vi "FV-View-R140_txt_multifile.vi"() -> ()   [LabVIEW 2020, in "FV-file_viewer.lvlib"]
uses:
  FV-file_viewer.lvlib
  record_file_handler/VFH-VNA_File_Handler.lvlib
  features/CF-common_features.lvlib
panel:
  out "All Files in Dir":path[](array[path])
  in  "Tab Control":enum32{"Page 1", "Page 3", "Page 2"}(tab)
  in  "Max range":dbl format="%#_6p"
  in  "min range":dbl format="%#_6p"
  out "Ref R":cluster{"Frequency":dbl[], "S21_Imag":dbl[]}[](graph)
  out "Ref I":cluster{"Frequency":dbl[], "S21_Imag":dbl[]}[](graph)
  out "p'":cluster{"Frequency":dbl[], "S21_Imag":dbl[]}[](graph)
  out "p''":cluster{"Frequency":dbl[], "S21_Imag":dbl[]}[](graph)
  in  "Stop":bool
  in  "Max range 2":dbl
  in  "min range 2":dbl
  out "Tan":cluster{"Frequency":dbl[], "S21_Imag":dbl[]}[](graph)
  out "Q [S/m]":cluster{"Frequency":dbl[], "S21_Imag":dbl[]}[](graph)
  in  "Stop 2":bool
  out "appended path":path
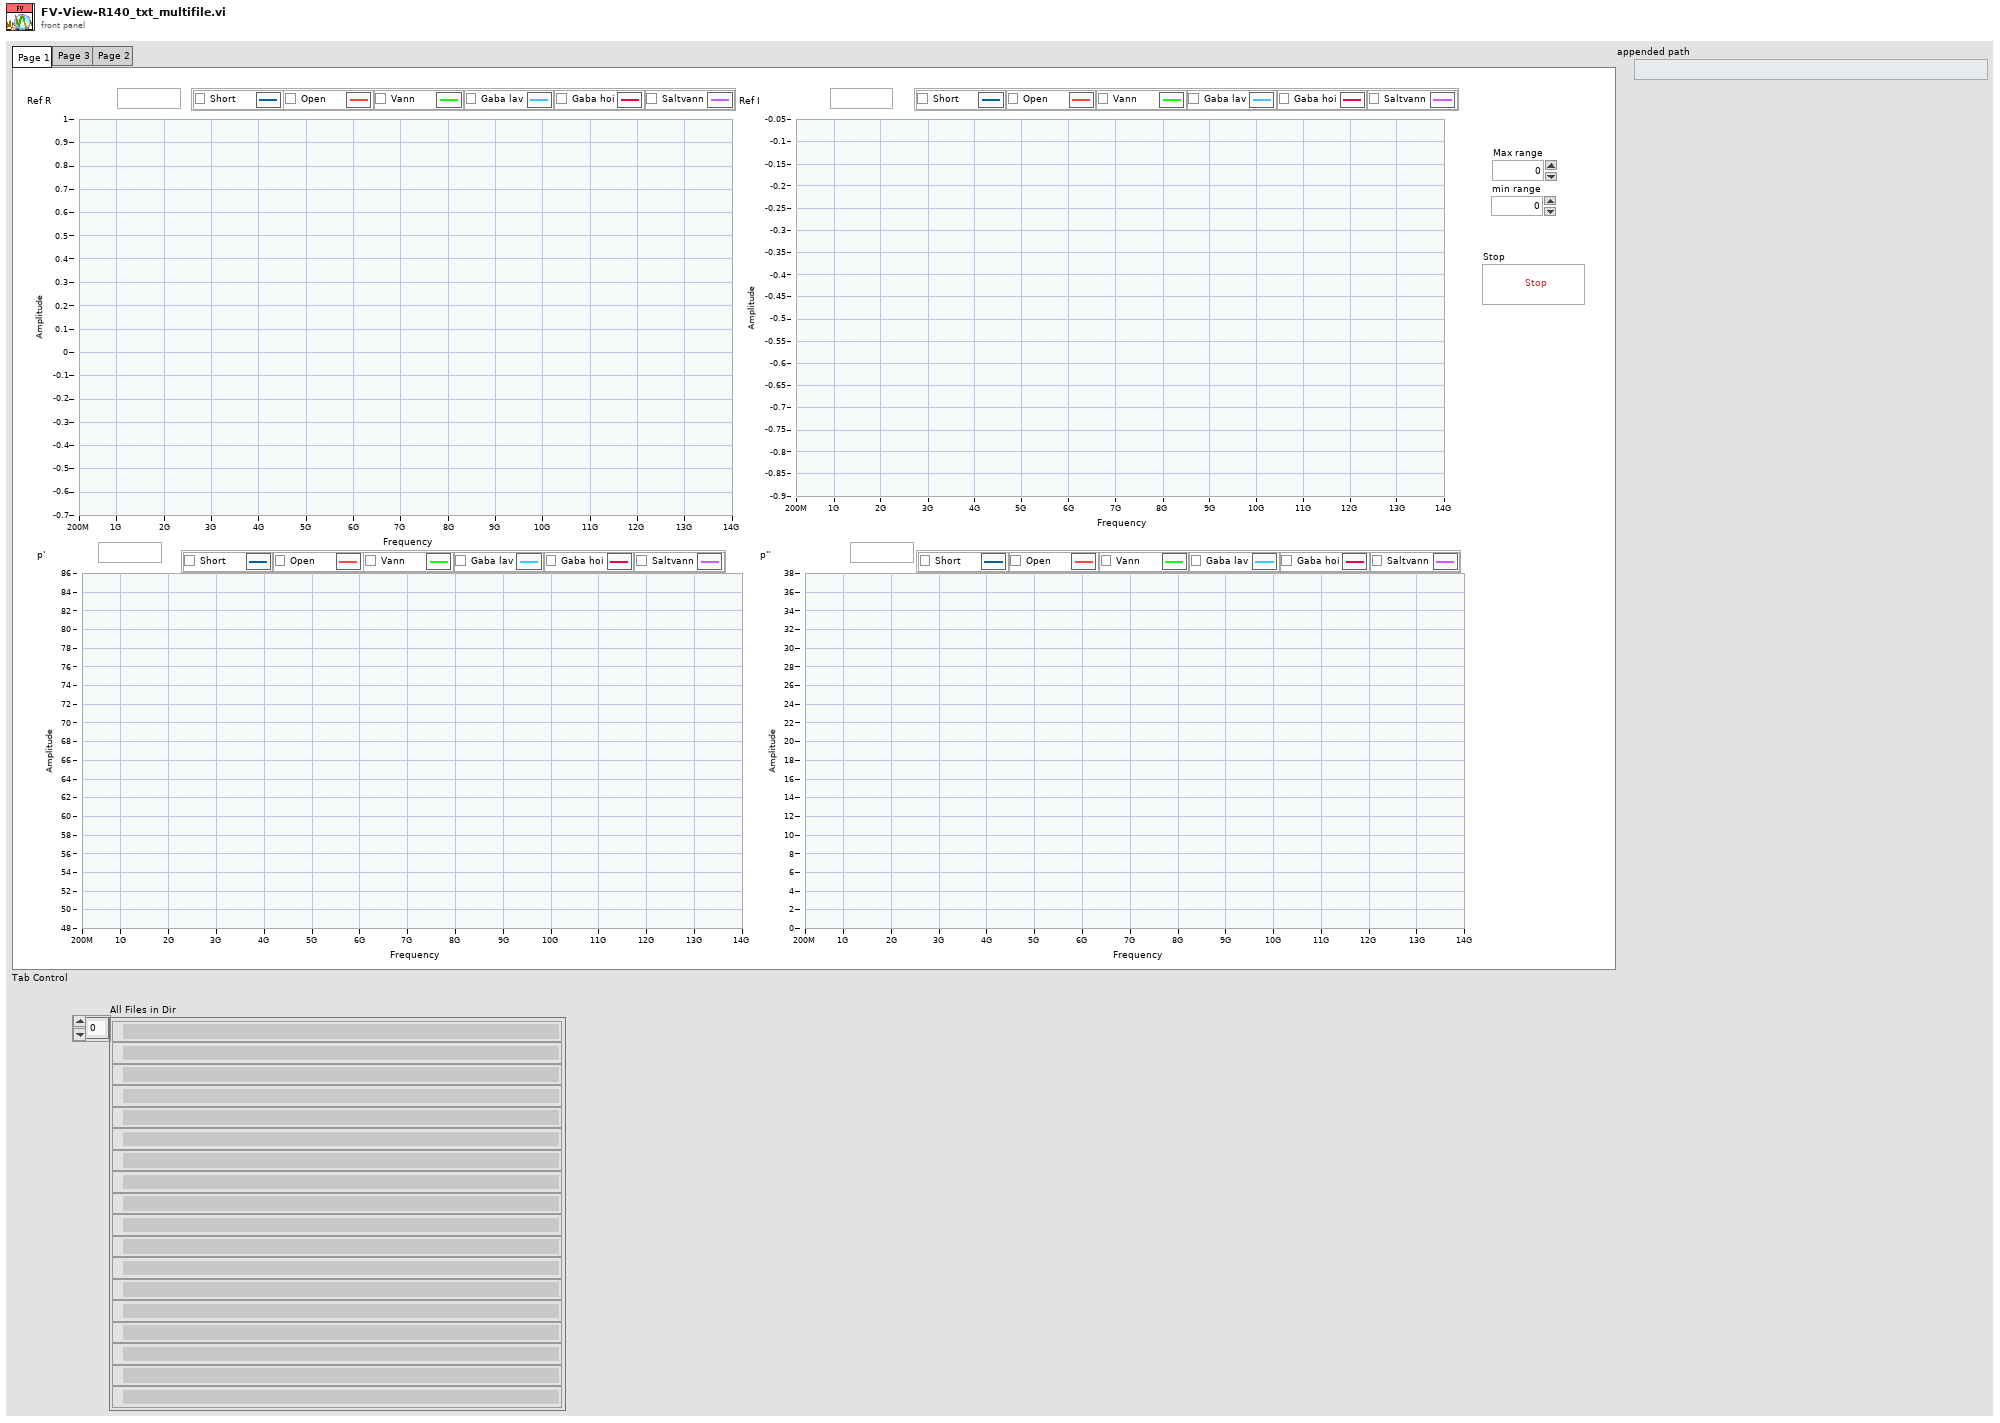
[diagram p1: front panel]
types:
  T1 = typedef "VFH-VNA_File_Handler.lvlib/VFH-file_cluster-LabVIEWVNA.ctl" = cluster{"Frequency":dbl[], "S1_Real":dbl[], "S1_Imag":dbl[], "S11_Real":dbl[], "S11_Imag":dbl[], "S21_Real":dbl[], "S21_Imag":dbl[]}
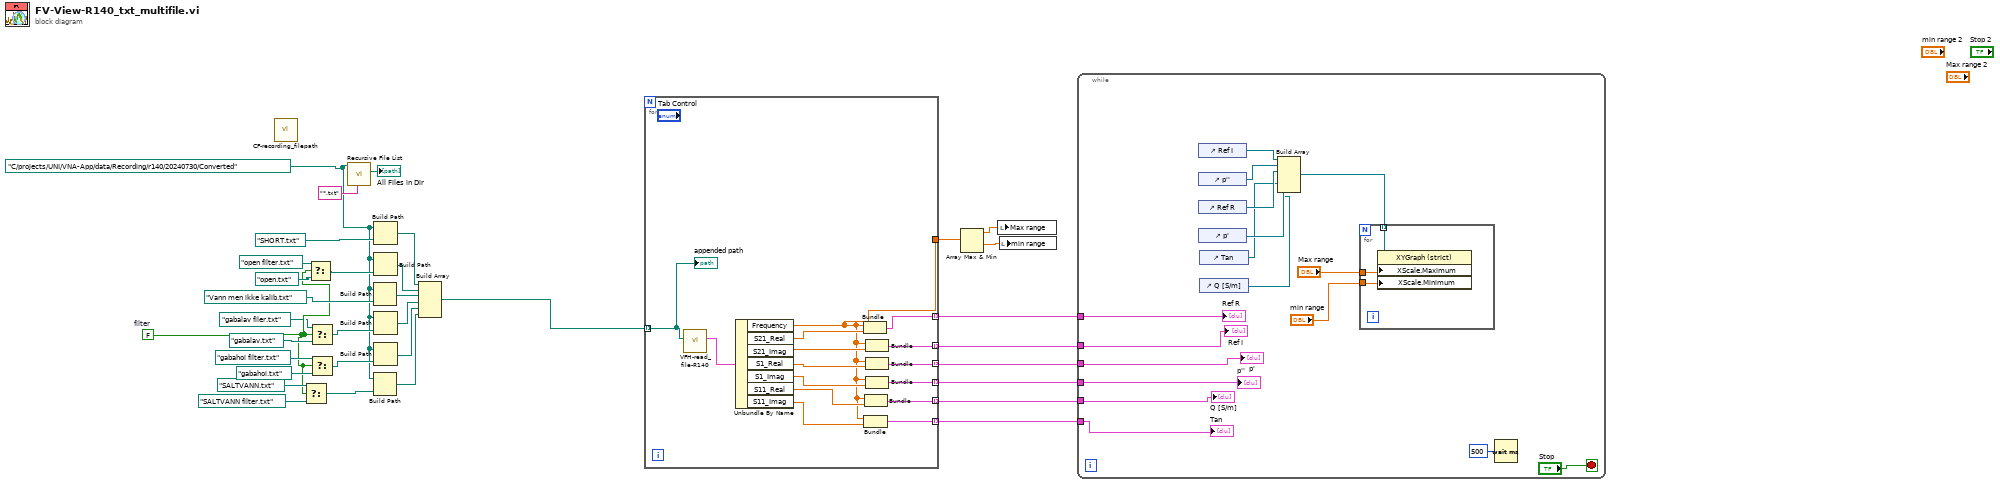
[diagram p0: block diagram]
diagram:
  w6 = FALSE  # filter
  w1 = path "C:/projects/UNI/VNA-App/data/Recording/r140/20240730/Converted" ("Folder Path")
  n1 = call "CF-recording_filepath.vi"() -> ()  [unwired: 10 in, 2 out]
  n2 = Select(t=path "SALTVANN.txt" ("name or relative path"), s=w6, f=path "SALTVANN filter.txt" ("name or relative path")) -> (s? t:f=w10:path)
  n3 = Select(t=path "open filter.txt" ("name or relative path"), s=w6, f=path "open.txt" ("name or relative path")) -> (s? t:f=w8:path)
  n4 = Select(t=path "gabalav filer.txt" ("name or relative path"), s=w6, f=path "gabalav.txt" ("name or relative path")) -> (s? t:f=w5:path)
  n5 = Select(t=path "gabahoi filter.txt" ("name or relative path"), s=w6, f=path "gabahoi.txt" ("name or relative path")) -> (s? t:f=w13:path)
  n6 = call <vilib>:"Recursive File List.vi"("pattern"="*.txt", "Folder Path"=w1) -> ("All Files in Dir"=→"All Files in Dir":path[])  [unwired: 5 in, 4 out]
  n7 = Build Path(base path=w1, name or relative path=path "Vann men ikke kalib.txt") -> (appended path=w23:path)
  n8 = Build Path(base path=w1, name or relative path=w10) -> (appended path=w20:path)
  n9 = Build Path(base path=w1, name or relative path=path "SHORT.txt") -> (appended path=w25:path)
  n10 = Build Path(base path=w1, name or relative path=w8) -> (appended path=w24:path)
  n11 = Build Path(base path=w1, name or relative path=w5) -> (appended path=w22:path)
  n12 = Build Path(base path=w1, name or relative path=w13) -> (appended path=w21:path)
  n13 = Build Array(w25, w24, w23, w22, w21, w20) -> (w18:path[])
  n14 = for {
    tunnel: w18 -> [w36] mode=indexing
    tunnel: [w45] -> w34 mode=indexing
    tunnel: [w44] -> w33 mode=indexing
    tunnel: [w43] -> w32 mode=indexing
    tunnel: [w42] -> w31 mode=indexing
    tunnel: [w39] -> w30
    tunnel: [w38] -> w27 mode=indexing
    tunnel: [w37] -> w26 mode=indexing
    n15 = call "VFH-read_file-R140.vi"("file path (dialog if empty)"=w36) -> ("output cluster"=w35:T1)  [unwired: 9 in, 1 out]
    n16 = Unbundle By Name(w35) -> ("Frequency"=w39:dbl[], "S21_Real"=w49:dbl[], "S21_Imag"=w48:dbl[], "S1_Real"=w47:dbl[], "S1_Imag"=w46:dbl[], "S11_Real"=w40:dbl[], "S11_Imag"=w41:dbl[])
    n17 = Bundle("Frequency"=w39, "S21_Real"=w49) -> (w45:cluster{"Frequency":dbl[], "S21_Real":dbl[]})  [unwired: 1 in]
    n18 = Bundle("Frequency"=w39, "S11_Imag"=w41) -> (w37:cluster{"Frequency":dbl[], "S11_Imag":dbl[]})  [unwired: 1 in]
    n19 = Bundle("Frequency"=w39, "S11_Real"=w40) -> (w38:cluster{"Frequency":dbl[], "S11_Real":dbl[]})  [unwired: 1 in]
    n20 = Bundle("Frequency"=w39, "S21_Imag"=w48) -> (w44:cluster{"Frequency":dbl[], "S21_Imag":dbl[]})  [unwired: 1 in]
    n21 = Bundle("Frequency"=w39, "S1_Real"=w47) -> (w43:cluster{"Frequency":dbl[], "S1_Real":dbl[]})  [unwired: 1 in]
    n22 = Bundle("Frequency"=w39, "S1_Imag"=w46) -> (w42:cluster{"Frequency":dbl[], "S1_Imag":dbl[]})  [unwired: 1 in]
    "appended path" <- w36
  }
  n23 = Array Max & Min(array=w30) -> (max value=w29:dbl, min value=w28:dbl)  [unwired: 2 out]
  n24 = local write "Max range"(w29) -> ()
  n25 = local write "min range"(w28) -> ()
  n26 = while {
    tunnel: w34 -> [w64]
    tunnel: w33 -> [w63]
    tunnel: w32 -> [w62]
    tunnel: w31 -> [w61]
    tunnel: w27 -> [w53]
    tunnel: w26 -> [w52]
    stop <- "Stop" stop-if-true
    n27 = control-ref of="Ref I"() -> (w60:refnum<vi>)
    n28 = control-ref of="p''"() -> (w59:refnum<vi>)
    n29 = control-ref of="Ref R"() -> (w58:refnum<vi>)
    n30 = control-ref of="p'"() -> (w57:refnum<vi>)
    n31 = control-ref of="Tan"() -> (w51:refnum<vi>)
    n32 = control-ref of="Q [S/m]"() -> (w50:refnum<vi>)
    n33 = Build Array(w60, w59, w58, w57, w51, w50) -> (w56:refnum<vi>[])
    n34 = for {
      tunnel: w56 -> [w69] mode=indexing
      tunnel: "Max range" -> [w68]
      tunnel: "min range" -> [w67]
      n35 = property class="XYGraph (strict)"(reference=w69, "XScale.Maximum"=w68, "XScale.Minimum"=w67) -> ()  [unwired: 1 in, 2 out]
    }
    n36 = Wait (ms)(milliseconds to wait=u32 500) -> ()  [unwired: 1 out]
    "p'" <- w62
    "Ref R" <- w64
    "p''" <- w61
    "Ref I" <- w63
    "Q [S/m]" <- w53
    "Tan" <- w52
  }
